vi "USB2XXX_LINEX_MasterLDFWriteRead.vi"() -> ()   [LabVIEW 2010]
panel:
  out "return type":i32
  in  "pValueStr 4":string
  out "iStARS_Voltage":string
  in  "pValueStr 3":string
  out "Exc_Current":string
  in  "pValueStr 2":string
  out "Exc_Duty_Cycle":string
  in  "Reg_Blind":dbl=1.0
  in  "MM_Request":dbl=2.0
  in  "Derat_Shift":dbl=2.0
  in  "Exc_Limitation":dbl=15.6
  in  "Cut_Off_Speed":dbl=4.0
  in  "Ramp_Time":dbl=3.0
  in  "Reg_Set_Voltage":dbl=13.5
  in  "pValueStr":string
  out "MM_State":string
  in  "pLDFFileName":string="example.ldf"
  in  "stop":bool
  in  "Channel Index":u8(ring) items=["LIN1", "LIN2"]
  in  "Device Index":i32(ring) items=["0", "1", "2", "3", "4", "5"]
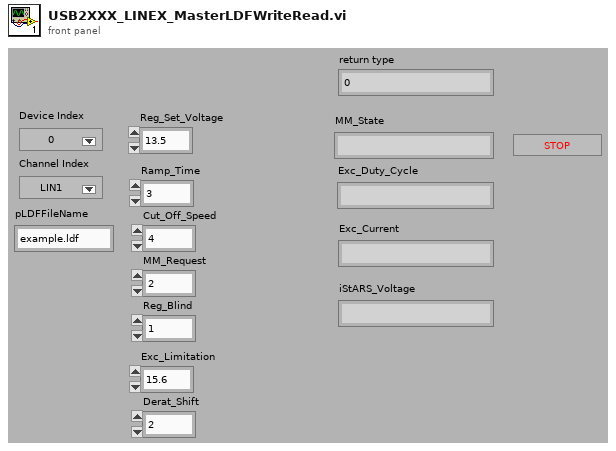
[diagram p1: front panel]
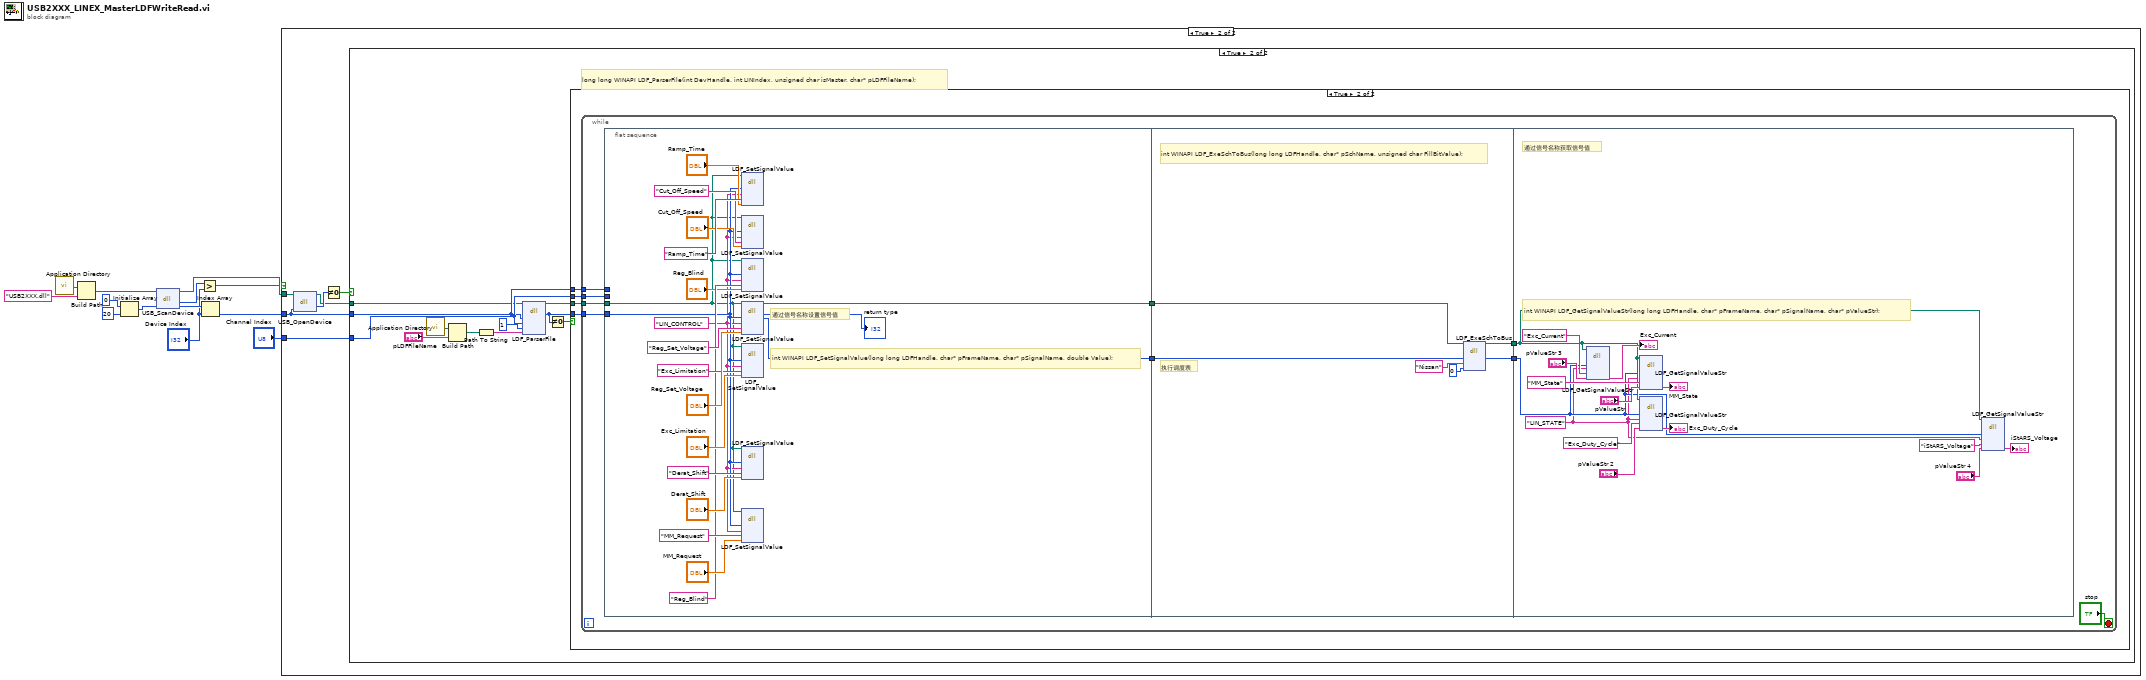
[diagram p0: block diagram]
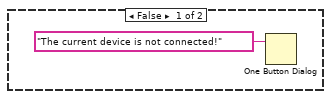
[diagram p2: hidden frame]
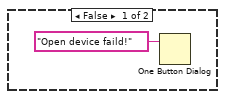
[diagram p3: hidden frame]
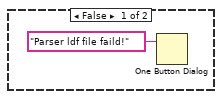
[diagram p4: hidden frame]
diagram:
  n1 = call <vilib>:"Application Directory.vi"() -> ("Application Directory"=w5:path)
  n2 = Build Path(base path=w5, name or relative path="USB2XXX.dll") -> (appended path=w4:path)
  n3 = Initialize Array(0, 20 ("dimension size")) -> (w11:i32[])
  n4 = dll-call lib="E:/OtherWork/STM32/USB2XXX_Example/examples/Labview/PublicFiles/USB2XXX.dll" fn="USB_ScanDevice"(path in=w4, "pDevNum"=w11) -> (path out=w9:path, "return type"=w3:i32, "pDevNum"=w10:i32[])  [unwired: 2 in, 1 out]
  n5 = Greater?(x=w3, y="Device Index") -> (0:w1:bool)
  n6 = Index Array(array=w10, index="Device Index") -> (element=w8:i32)
  n7 = case shown="True" w1 {
    tunnel: w9 -> [_ w20]
    tunnel: w8 -> [_ w16]
    tunnel: "Channel Index" -> [_ w15]
    frame False {
      n8 = One Button Dialog(message="The current device is not connected!") -> ()  [unwired: 1 in, 1 out]
    }
    frame True {
      n9 = dll-call lib="E:/OtherWork/STM32/USB2XXX_Example/examples/Labview/PublicFiles/USB2XXX.dll" fn="USB_OpenDevice"(path in=w20, "DevIndex"=w16) -> (path out=w17:path, "return type"=w19:u8)  [unwired: 3 in, 1 out]
      n10 = Not Equal To 0?(x=w19) -> (x != 0?=w18:bool)
      n11 = case shown="True" w18 {
        tunnel: w17 -> [_ w28]
        tunnel: w16 -> [_ w30]
        tunnel: w15 -> [_ w31]
        frame False {
          n12 = One Button Dialog(message="Open device faild!") -> ()  [unwired: 1 in, 1 out]
        }
        frame True {
          # "long long WINAPI LDF_ParserFile(int DevHandle, int LINIndex, unsigned char isMaster, char* pLDFFileName);"
          n13 = call <vilib>:"Application Directory.vi"() -> ("Application Directory"=w25:path)
          n14 = Build Path(base path=w25, name or relative path="pLDFFileName") -> (appended path=w23:path)
          n15 = Path To String(path=w23) -> (string=w22:string)
          n16 = dll-call lib="E:/Projects/USB2XXX/trunk/USB2XXX/USB2XXX/vs2019/Release/USB2XXX.*" fn="LDF_ParserFile"(path in=w28, "DevHandle"=w30, "LINIndex"=w31, "isMaster"=u8 1, "pLDFFileName"=w22) -> (path out=w29:path, "return type"=w26:u64)  [unwired: 6 in, 1 out]
          n17 = Not Equal To 0?(x=w26) -> (x != 0?=w27:bool)
          n18 = case shown="True" w27 {
            tunnel: w29 -> [_ w37]
            tunnel: w30 -> [_ w36]
            tunnel: w31 -> [_ w35]
            tunnel: w26 -> [_ w34]
            frame False {
              n19 = One Button Dialog(message="Parser ldf file faild!") -> ()  [unwired: 1 in, 1 out]
            }
            frame True {
              n20 = while {
                tunnel: w37 -> [w46]
                tunnel: w36 -> [w45]
                tunnel: w35 -> [w44]
                tunnel: w34 -> [w42]
                stop <- "stop" stop-if-true
                n21 = flat-sequence {
                  tunnel: w46 -> [w50]
                  tunnel: w45 -> [_]
                  tunnel: w44 -> [_]
                  tunnel: w42 -> [w52]
                  tunnel: [w49] -> w41
                  tunnel: [w48] -> w40
                  tunnel: w41 -> [w72]
                  tunnel: w40 -> [w68]
                  tunnel: [w67] -> w39
                  tunnel: [w69] -> w38
                  tunnel: w39 -> [w75]
                  tunnel: w38 -> [w74]
                  frame #0 {
                    w51 = "LIN_CONTROL" ("pFrameName")
                    # "int WINAPI LDF_SetSignalValue(long long LDFHandle, char* pFrameName, char* pSignalName, double Value);"
                    # "通过信号名称设置信号值"
                    n22 = dll-call lib="E:/Projects/USB2XXX/trunk/USB2XXX/USB2XXX/vs2019/Release/USB2XXX.*" fn="LDF_SetSignalValue"(path in=w50, "LDFHandle"=w52, "pFrameName"=w51, "pSignalName"="Ramp_Time", "Value"="Ramp_Time") -> ()  [unwired: 7 in, 2 out]
                    n23 = dll-call lib="E:/Projects/USB2XXX/trunk/USB2XXX/USB2XXX/vs2019/Release/USB2XXX.*" fn="LDF_SetSignalValue"(path in=w50, "LDFHandle"=w52, "pFrameName"=w51, "pSignalName"="Cut_Off_Speed", "Value"="Cut_Off_Speed") -> ()  [unwired: 7 in, 2 out]
                    n24 = dll-call lib="E:/Projects/USB2XXX/trunk/USB2XXX/USB2XXX/vs2019/Release/USB2XXX.*" fn="LDF_SetSignalValue"(path in=w50, "LDFHandle"=w52, "pFrameName"=w51, "pSignalName"="Reg_Blind", "Value"="Reg_Blind") -> ()  [unwired: 7 in, 2 out]
                    n25 = dll-call lib="E:/Projects/USB2XXX/trunk/USB2XXX/USB2XXX/vs2019/Release/USB2XXX.*" fn="LDF_SetSignalValue"(path in=w50, "LDFHandle"=w52, "pFrameName"=w51, "pSignalName"="Reg_Set_Voltage", "Value"="Reg_Set_Voltage") -> (path out=w48:path, "return type"=→"return type":i32, "LDFHandle"=w49:u64)  [unwired: 5 in, 1 out]
                    n26 = dll-call lib="E:/Projects/USB2XXX/trunk/USB2XXX/USB2XXX/vs2019/Release/USB2XXX.*" fn="LDF_SetSignalValue"(path in=w50, "LDFHandle"=w52, "pFrameName"=w51, "pSignalName"="Exc_Limitation", "Value"="Exc_Limitation") -> ()  [unwired: 7 in, 2 out]
                    n27 = dll-call lib="E:/Projects/USB2XXX/trunk/USB2XXX/USB2XXX/vs2019/Release/USB2XXX.*" fn="LDF_SetSignalValue"(path in=w50, "LDFHandle"=w52, "pFrameName"=w51, "pSignalName"="Derat_Shift", "Value"="Derat_Shift") -> ()  [unwired: 7 in, 2 out]
                    n28 = dll-call lib="E:/Projects/USB2XXX/trunk/USB2XXX/USB2XXX/vs2019/Release/USB2XXX.*" fn="LDF_SetSignalValue"(path in=w50, "LDFHandle"=w52, "pFrameName"=w51, "pSignalName"="MM_Request", "Value"="MM_Request") -> ()  [unwired: 7 in, 2 out]
                  }
                  frame #1 {
                    # "int WINAPI LDF_ExeSchToBus(long long LDFHandle, char* pSchName, unsigned char FillBitValue);"
                    # "执行调度表"
                    n29 = dll-call lib="E:/Projects/USB2XXX/trunk/USB2XXX/USB2XXX/vs2019/Release/USB2XXX.*" fn="LDF_ExeSchToBus"(path in=w68, "LDFHandle"=w72, "pSchName"="Nissan", "FillBitValue"=u8 0) -> (path out=w67:path, "LDFHandle"=w69:u64)  [unwired: 5 in, 1 out]
                  }
                  frame #2 {
                    w73 = "LIN_STATE" ("pFrameName")
                    # "int WINAPI LDF_GetSignalValueStr(long long LDFHandle, char* pFrameName, char* pSignalName, char* pValueStr);"
                    # "通过信号名称获取信号值"
                    n30 = dll-call lib="E:/Projects/USB2XXX/trunk/USB2XXX/USB2XXX/vs2019/Release/USB2XXX.*" fn="LDF_GetSignalValueStr"(path in=w75, "LDFHandle"=w74, "pFrameName"=w73, "pSignalName"="Exc_Current", "pValueStr"="pValueStr 3") -> ("pValueStr"=→"Exc_Current":string)  [unwired: 6 in, 2 out]
                    n31 = dll-call lib="E:/Projects/USB2XXX/trunk/USB2XXX/USB2XXX/vs2019/Release/USB2XXX.*" fn="LDF_GetSignalValueStr"(path in=w75, "LDFHandle"=w74, "pFrameName"=w73, "pSignalName"="MM_State", "pValueStr"="pValueStr") -> ("pValueStr"=→"MM_State":string)  [unwired: 6 in, 2 out]
                    n32 = dll-call lib="E:/Projects/USB2XXX/trunk/USB2XXX/USB2XXX/vs2019/Release/USB2XXX.*" fn="LDF_GetSignalValueStr"(path in=w75, "LDFHandle"=w74, "pFrameName"=w73, "pSignalName"="Exc_Duty_Cycle", "pValueStr"="pValueStr 2") -> ("pValueStr"=→"Exc_Duty_Cycle":string)  [unwired: 6 in, 2 out]
                    n33 = dll-call lib="E:/Projects/USB2XXX/trunk/USB2XXX/USB2XXX/vs2019/Release/USB2XXX.*" fn="LDF_GetSignalValueStr"(path in=w75, "LDFHandle"=w74, "pFrameName"=w73, "pSignalName"="iStARS_Voltage", "pValueStr"="pValueStr 4") -> ("pValueStr"=→"iStARS_Voltage":string)  [unwired: 6 in, 2 out]
                  }
                }
              }
            }
          }
        }
      }
    }
  }
